vi "CMC_Homework_05.vi"() -> ()   [LabVIEW 2013]
panel:
  out "XY Graph":cluster{dbl[], dbl[]}[](graph)
  in  "Table Control":string[][](table)
  # "In Collaboration with Sarah Bailey & Alex Ofredi"
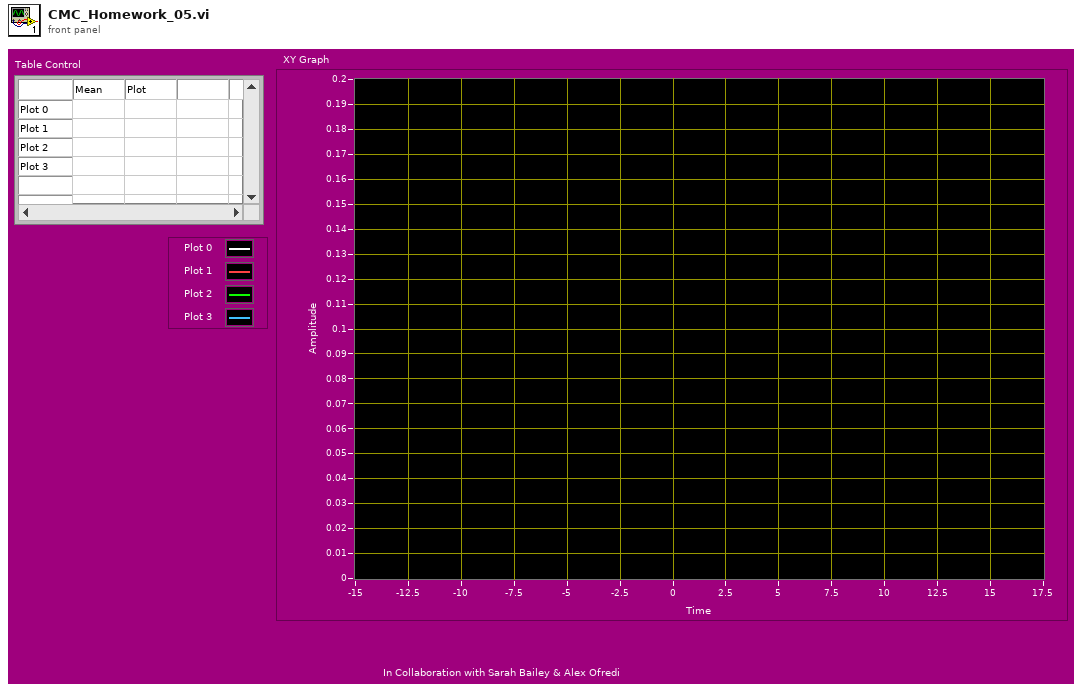
[diagram p1: front panel]
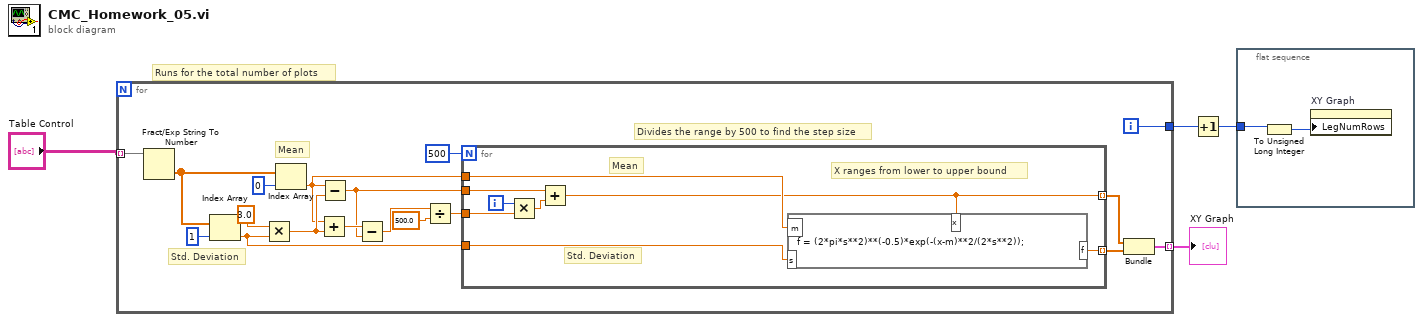
[diagram p0: block diagram]
diagram:
  # "Runs for the total number of plots"
  n1 = for {
    tunnel: "Table Control" -> [w18] mode=indexing
    tunnel: [w6] -> w4 mode=indexing
    tunnel: [w5] -> w2
    i -> [w5]
    # "Divides the range by 500 to find the step size"
    # "Std. Deviation"
    # "Mean"
    n2 = Fract/Exp String To Number(string=w18) -> (number=w17:dbl[])  [unwired: 3 in, 1 out]
    n3 = Index Array(array=w17, index=1) -> (element=w9:dbl)
    n4 = Multiply(x=3.0, y=w9) -> (x*y=w15:dbl)
    n5 = Index Array(array=w17, index=0) -> (element=w8:dbl)
    n6 = Add(x=w8, y=w15) -> (x+y=w14:dbl)
    n7 = Subtract(x=w8, y=w15) -> (x-y=w7:dbl)
    n8 = Subtract(x=w14, y=w7) -> (x-y=w12:dbl)
    n9 = Divide(x=w12, y=500.0) -> (x/y=w10:dbl)
    n10 = for {
      N: 500 -> [_]
      tunnel: [w30] -> w22 mode=indexing
      tunnel: [w23] -> w21 mode=indexing
      tunnel: w9 -> [w29]
      tunnel: w8 -> [w28]
      tunnel: w10 -> [w27]
      tunnel: w7 -> [w24]
      i -> [w26]
      # "Mean"
      # "Std. Deviation"
      # "X ranges from lower to upper bound"
      n11 = Multiply(x=w26, y=w27) -> (x*y=w25:dbl)
      n12 = Add(x=w24, y=w25) -> (x+y=w23:dbl)
      n13 = formula code="f = (2*pi*s**2)**(-0.5)*exp(-(x-m)**2/(2*s**2));"("s"=w29, "m"=w28, "x"=w23) -> ("f"=w30:dbl)
    }
    n14 = Bundle(w21, w22) -> (w6:cluster{dbl[], dbl[]})  [unwired: 1 in]
  }
  "XY Graph" <- w4
  n15 = Increment(x=w2) -> (x+1=w3:i32)
  n16 = flat-sequence {
    tunnel: w3 -> [w31]
    frame #0 {
      n17 = To Unsigned Long Integer(number=w31) -> (unsigned 32bit integer=w32:u32)
      n18 = property on="XY Graph" class="XYGraph (strict)"("LegNumRows"=w32) -> ()  [unwired: 2 in, 2 out]
    }
  }
